vi "污染物CP编码.vi"(6 "字符串":string="N", 7 "字段结束":bool=TRUE, 8 "数据类型":string(combo)="-Rtd=", 9 "污染物浓度":string, 10 "污染物编码":string) -> (3 "编码输出":string)   [LabVIEW 2016, in "数据传输系统.lvlib"]
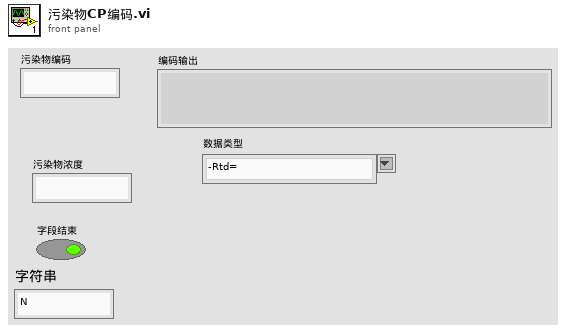
[diagram p1: front panel]
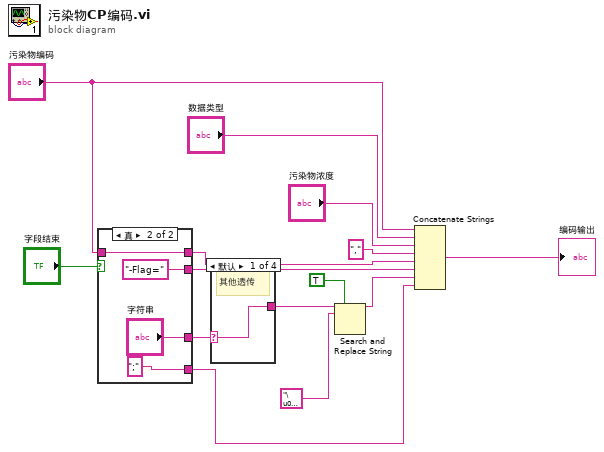
[diagram p0: block diagram]
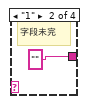
[diagram p2: hidden frame]
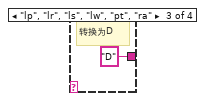
[diagram p3: hidden frame]
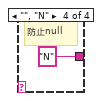
[diagram p4: hidden frame]
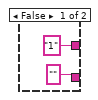
[diagram p5: hidden frame]
diagram:
  n1 = case shown="真" "字段结束" {
    tunnel: [_ "-Flag=" ("字符串")] -> w10
    tunnel: ["1" ("字符串") "字符串"] -> w6
    tunnel: "污染物编码" -> [_ w19]
    tunnel: [_ w19] -> w7
    tunnel: ["" ("字符串") ";" ("字符串")] -> w1
    frame False {
    }
    frame True {
    }
  }
  n2 = case shown="默认" w6 {
    selector: w6 -> [w21 _ _ _]
    tunnel: [w21 "" ("字符串") "D" ("字符串") "N" ("字符串")] -> w5
    frame Default {
      # "其他透传"
    }
    frame "1" {
      # "字段未完"
    }
    frame "lp", "lr", "ls", "lw", "pt", "ra" {
      # "转换为D"
    }
    frame "", "N" {
      # "防止null"
    }
  }
  n3 = Search and Replace String(replace all?=TRUE ("替换全部？(F)"), input string=w5, search string="\u0000" ("搜索字符串")) -> (result string=w3:string)  [unwired: 5 in, 3 out]
  n4 = Concatenate Strings("污染物编码", "数据类型", "污染物浓度", "," ("字符串"), w7, w10, w3, w1) -> (→"编码输出":string)
